vi "PipelineDuty.vi"(8 "error in (no error)":errorcluster, 10 "DataExchange":T1, 11 "GRMActor in":refnum<class "StageController.lvclass">) -> (0 "error out":errorcluster, 2 "DataExchange Out":T1, 3 "GRMActor out":refnum<class "StageController.lvclass">)   [LabVIEW 2020]
uses:
  Model/Hardware Abstraction Layer/Component/Device/Device/DataExchange.ctl
  Interface/DataListener/DataListener.lvclass
  StageController.lvclass
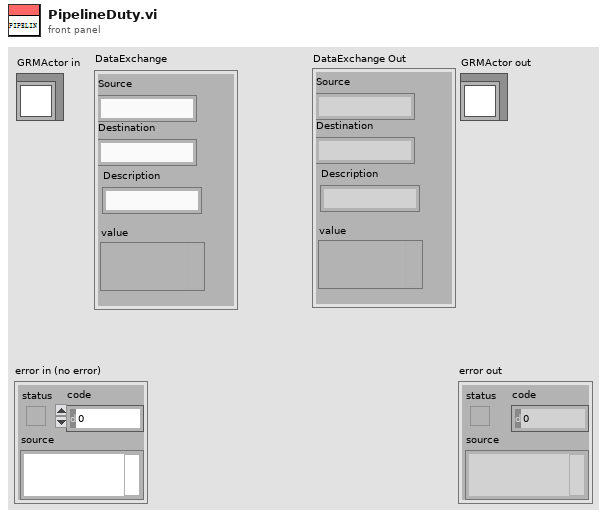
[diagram p1: front panel]
types:
  T1 = typedef "DataListener.lvclass/DataExchange.ctl" = cluster{"Source":string, "Destination":string, "Description":string, "value":variant}
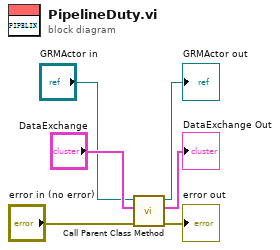
[diagram p0: block diagram]
diagram:
  n1 = call-parent "Call Parent Class Method"("error in (no error)"="error in (no error)", "DataExchange"="DataExchange", "GRMActor in"="GRMActor in") -> ("error out"=→"error out":errorcluster, "DataExchange Out"=→"DataExchange Out":T1, "GRMActor out"=→"GRMActor out":refnum<class "StageController.lvclass">)  [unwired: 6 in]
